vi "Find Post-Setup Actors.vi"(9 "Composed Actor":refnum<class "Actor.lvclass">, 10 "Actor":refnum<class "Actor.lvclass">) -> (2 "Post-Setup Actors":refnum<class "Actor.lvclass">[](array[class]))   [LabVIEW 2020, in "jettl.lvlib"]
uses:
  jettl.lvlib
  Actor/Actor.lvclass
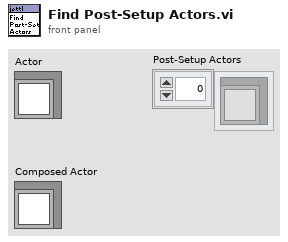
[diagram p1: front panel]
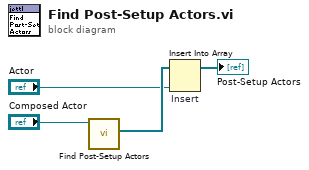
[diagram p0: block diagram]
diagram:
  n1 = call-dynamic "Find Post-Setup Actors.vi"("Actor in"="Composed Actor") -> ("Post-Setup Actors"=w3:refnum<class "Actor.lvclass">[])  [unwired: 10 in]
  n2 = Insert Into Array "Insert"(array=w3, new element="Actor") -> (→"Post-Setup Actors":refnum<class "Actor.lvclass">[])  [unwired: 1 in]
